vi "build token URI.vi"(8 "error in (no error)":errorcluster, 11 "Oauth2.LinkedIn in":refnum<class "Oauth2.LinkedIn.lvclass">) -> (0 "error out":errorcluster, 1 "Headers":cluster{"header":string, "value":string}[](array[cluster]), 2 "Token Request URI":string, 3 "Oauth2.LinkedIn":refnum<class "Oauth2.LinkedIn.lvclass">)   [LabVIEW 2017, in "Oauth2.LinkedIn.lvclass"]
uses:
  Oauth2.LinkedIn.lvclass
  D:/GitHub/Oauth2/source/Oauth2/Oauth2.lvclass
  OAuthToken/OAuth2 Token Element -- enum.ctl
  Oauth2/Oauth2.lvclass/Oauth2.ctl
  <vilib>/LabVIEW Open Source Project/OpenURI/uri/URI.lvclass
  OAuthToken/OAuthAccessToken.lvclass
  Oauth2/Oauth2.lvclass
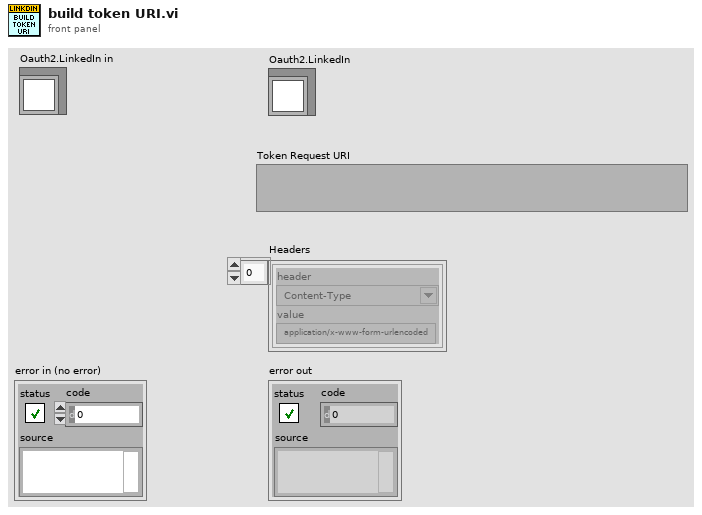
[diagram p1: front panel]
types:
  T1 = typedef "OAuthAccessToken.lvclass/OAuth2 Token Element -- enum.ctl" = enum16{"client_id", "client_secret", "response_type", "scope", "redirect_uri", "error", "error_description", "error_uri", "grant_type", "code", "access_token", "token_type", "expires_in", "username", "password", "refresh_token", "code_challenge", "code_challenge_method", "reverse_proxy_uri", "endpoint element", "prompt", "access_type", "id_token"}
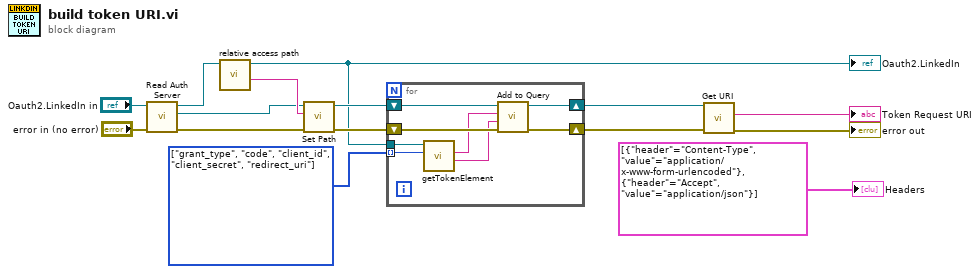
[diagram p0: block diagram]
diagram:
  w7 = T1[] [enum."grant_type", enum."code", enum."client_id", enum."client_secret", enum."redirect_uri"] items=["client_id", "client_secret", "response_type", "scope", "redirect_uri", "error", "error_description", "error_uri", "grant_type", "code", "access_token", "token_type", "expires_in", "username", "password", "refresh_token", "code_challenge", "code_challenge_method", "reverse_proxy_uri", "endpoint element", "prompt", "access_type", "id_token"]
  n1 = call "Read Auth Server.vi"("error in (no error)"="error in (no error)", "Oauth2 in"="Oauth2.LinkedIn in") -> ("error out"=w2:errorcluster, "openURI.lvlib:URI.lvclass"=w3:refnum<class "URI.lvclass">, "Oauth2 out"=w4:refnum<class "Oauth2.LinkedIn.lvclass">)  [unwired: 7 in]
  "Oauth2.LinkedIn" <- w4
  n2 = call-dynamic "relative access path.vi"("Oauth2.LinkedIn"=w4) -> ("Token Access Path"=w10:string)  [unwired: 9 in, 1 out]
  n3 = call <vilib>:"Set Path.vi"("error in (no error)"=w2, "path"=w10, "URI in"=w3) -> ("error out"=w13:errorcluster, "URI out"=w14:refnum<class "URI.lvclass">)  [unwired: 7 in]
  n4 = for {
    shift-right: [w21] -> w9
    shift-left: w14 -> [w22]
    shift-right: [w19] -> w8
    shift-left: w13 -> [w20]
    tunnel: w4 -> [w18]
    tunnel: w7 -> [w16] mode=indexing
    n5 = call "getTokenElement.vi"("Token element"=w16, "Oauth2 in"=w18) -> ("Value"=w15:string, "Key"=w17:string)  [unwired: 5 in, 3 out]
    n6 = call <vilib>:"Add to Query.vi"("error in (no error)"=w20, "value"=w15, "key"=w17, "URI in"=w22) -> ("error out"=w19:errorcluster, "URI out"=w21:refnum<class "URI.lvclass">)  [unwired: 6 in]
  }
  n7 = call <vilib>:"Get URI.vi"("error in (no error)"=w8, "URI in"=w9) -> ("error out"=→"error out":errorcluster, "URI String"=→"Token Request URI":string)  [unwired: 7 in, 1 out]
  "Headers" <- cluster{"header":string, "value":string}[] [{"header"="Content-Type", "value"="application/x-www-form-urlencoded"}, {"header"="Accept", "value"="application/json"}] ("Headers")
